vi "Calibration Verifier using Simple State Machine.vi"() -> ()   [LabVIEW 2023]
uses:
  Agilent 3446X Series/Agilent 3446X Series.lvlib
  Keysight E36300 Series/Keysight E36300 Series.lvlib
panel:
  out "error out":errorcluster
  in  "error in":errorcluster
  out "Stabilization":u16(slide) scale=0.0..500.0
  out "Overall Verification":bool
  in  "Test Points & Results":T1(array[cluster])=[{"Volt Set Point (V)"=1.0, "Std Meas (V)"=0.0, "UUT Meas (V)"=0.0, "+/-Delta (V)"=0.1, "Result"=FALSE, "Error (mV)"=0.0}, {"Volt Set Point (V)"=3.3, "Std Meas (V)"=0.0, "UUT Meas (V)"=0.0, "+/-Delta (V)"=0.1, "Result"=FALSE, "Error (mV)"=0.0}, {"Volt Set Point (V)"=5.0, "Std Meas (V)"=0.0, "UUT Meas (V)"=0.0, "+/-Delta (V)"=0.1, "Result"=FALSE, "Error (mV)"=0.0}, {"Volt Set Point (V)"=10.0, "Std Meas (V)"=0.0, "UUT Meas (V)"=0.0, "+/-Delta (V)"=0.1, "Result"=FALSE, "Error (mV)"=0.0}, {"Volt Set Point (V)"=12.0, "Std Meas (V)"=0.0, "UUT Meas (V)"=0.0, "+/-Delta (V)"=0.1, "Result"=FALSE, "Error (mV)"=0.0}]
  # "Multimeter Calibration Verifier"
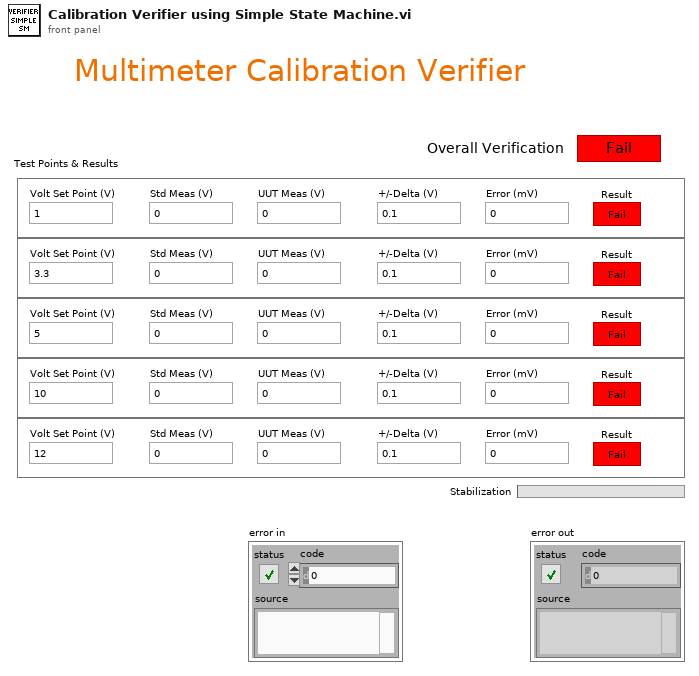
[diagram p1: front panel]
types:
  T1 = cluster{"Volt Set Point (V)":dbl, "Std Meas (V)":dbl, "UUT Meas (V)":dbl, "+/-Delta (V)":dbl, "Result":bool, "Error (mV)":dbl}[]
  T2 = enum16{"Start Calibration", "Set Volt to Power Supply", "Wait for stability", "Dialog Input UUT Meas", "Measure DMM", "Check Limits", "Update Overall Result", "Save Report"}
  T3 = cluster{"Volt Set Point (V)":dbl, "Std Meas (V)":dbl, "UUT Meas (V)":dbl, "+/-Delta (V)":dbl, "Result":bool, "Error (mV)":dbl}
  T4 = typedef "imagedata.ctl" = cluster{"image type":i32, "image depth":i32, "image":u8[], "mask":u8[], "colors":u32[], "Rectangle":cluster{"left":i16, "top":i16, "right":i16, "bottom":i16}}
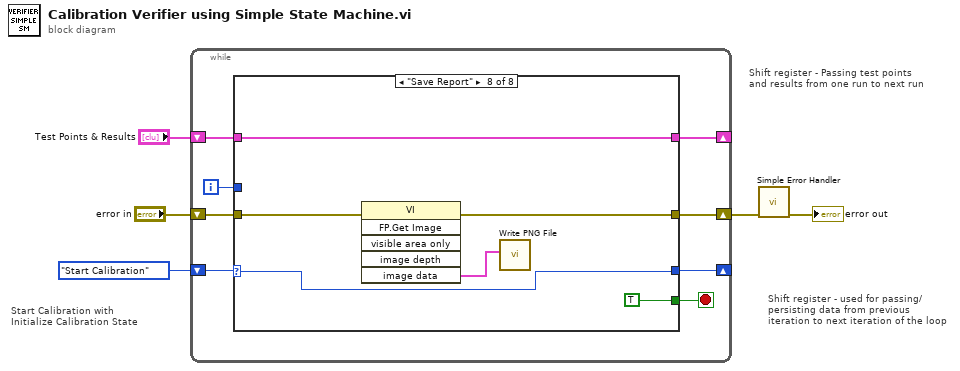
[diagram p0: block diagram]
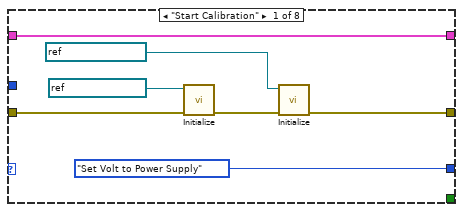
[diagram p2: hidden frame]
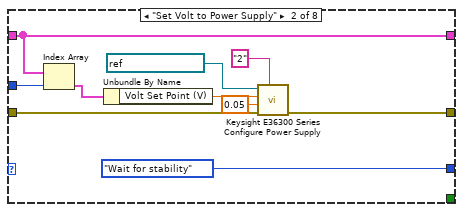
[diagram p3: hidden frame]
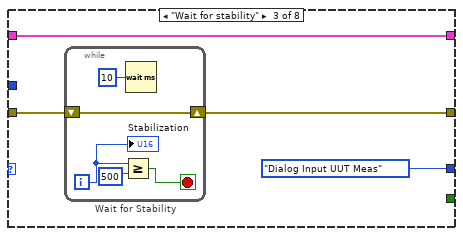
[diagram p4: hidden frame]
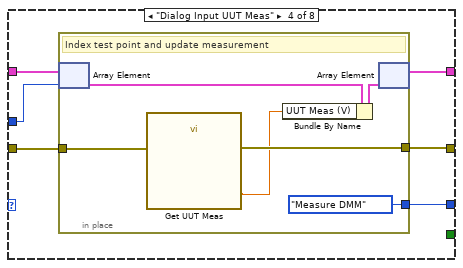
[diagram p5: hidden frame]
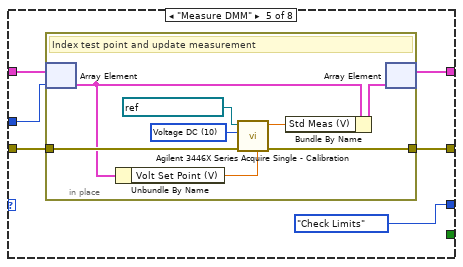
[diagram p6: hidden frame]
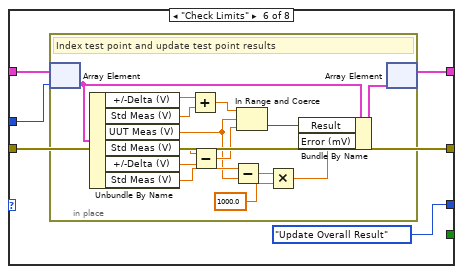
[diagram p7: hidden frame]
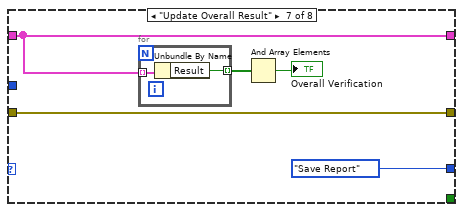
[diagram p8: hidden frame]
diagram:
  # "Shift register - Passing test points and results from one run to next run"
  # "Shift register - used for passing/persisting data from previous iteration to next iteration of the loop"
  # "Start Calibration with  Initialize Calibration State"
  n1 = while {
    shift-right: [w13] -> w4
    shift-left: "error in" -> [w12]
    shift-right: [w8] -> _
    shift-left: "Test Points & Results" -> [w7]
    shift-right: [w10] -> _
    shift-left: T2."Start Calibration" -> [w11]
    i -> [w6]
    stop <- w9 stop-if-true
    n2 = case shown="\"Save Report\"" w11 {
      selector: w11 -> [_ _ _ _ _ _ _ w95]
      tunnel: [w19 w24 w34 w44 w56 w70 w85 w92] -> w13
      tunnel: w12 -> [w18 w30 w31 w45 w57 w70 w85 w93]
      tunnel: [T2."Set Volt to Power Supply" T2."Wait for stability" T2."Dialog Input UUT Meas" w43 T2."Check Limits" T2."Update Overall Result" T2."Save Report" w95] -> w10
      tunnel: [_ _ _ _ _ _ _ TRUE] -> w9
      tunnel: w7 -> [w17 w23 w33 w42 w53 w68 w87 w96]
      tunnel: [w17 w23 w33 w40 w52 w67 w87 w96] -> w8
      tunnel: w6 -> [_ w22 _ w41 w54 w66 _ _]
      frame "Start Calibration" {
        n3 = call "Initialize.vi"("error in (no error)"=w18, "VISA resource name"=refnum<visa-resource-name> "E36312A_PSU") -> ("error out"=w20:errorcluster)  [unwired: 8 in, 1 out]
        n4 = call "Initialize.vi"("error in (no error)"=w20, "VISA resource name"=refnum<visa-resource-name> "34465A_DMM") -> ("error out"=w19:errorcluster)  [unwired: 8 in, 1 out]
      }
      frame "Set Volt to Power Supply" {
        n5 = Index Array(array=w23, index=w22) -> (element=w21:T3)
        n6 = Unbundle By Name(w21) -> ("Volt Set Point (V)"=w27:dbl)
        n7 = call "Keysight E36300 Series Configure Power Supply.vi"("Channel (1)"="2", "error in (no error)"=w30, "Current Level (2 A)"=0.05, "Voltage Level (1 V)"=w27, "VISA resource name"=refnum<visa-resource-name> "E36312A_PSU") -> ("error out"=w24:errorcluster)  [unwired: 6 in]
      }
      frame "Wait for stability" {
        n8 = while "Wait for Stability" {
          shift-right: [w35] -> w34
          shift-left: w31 -> [w35]
          i -> [w38]
          stop <- w36 stop-if-true
          n9 = Greater Or Equal?(x=w38, y=500) -> (x >= y?=w36:bool)
          n10 = Wait (ms)(milliseconds to wait=u32 10) -> ()  [unwired: 1 out]
          "Stabilization" <- w38
        }
      }
      frame "Dialog Input UUT Meas" {
        n11 = in-place {
          in-place-border: w45 -> [w51]
          in-place-border: [w50] -> w44
          in-place-border: [T2."Measure DMM"] -> w43
          # "Index test point and update measurement"
          n12 = in-place-array #1(w42, w41) -> (w46:T3)
          n13 = call "Get UUT Meas"("error in (no error)"=w51) -> ("Voltage (V)"=w49:dbl, "error out"=w50:errorcluster)  [unwired: 16 in, 1 out]
          n14 = Bundle By Name(cluster=w46, "UUT Meas (V)"=w49) -> (w47:T3)
          n15 = in-place-array #1(w47) -> (w40:T1)  [unwired: 1 out]
        }
      }
      frame "Measure DMM" {
        n16 = in-place {
          in-place-border: w57 -> [w65]
          in-place-border: [w64] -> w56
          w63 = 10 items=["Continuity", "Current AC", "Current DC", "Diode", "Frequency", "Resistance 4-wire", "Period", "Resistance 2-wire", "Temperature", "Voltage AC", "Voltage DC", "Voltage DC Ratio", "Capacitance"] ("Measurement Function (10: Voltage DC)")
          # "Index test point and update measurement"
          n17 = in-place-array #2(w53, w54) -> (w59:T3)
          n18 = Unbundle By Name(w59) -> ("Volt Set Point (V)"=w62:dbl)
          n19 = call "Agilent 3446X Series Acquire Single - Calibration.vi"("Sim. Volt Set Point (V)"=w62, "error in (no error)"=w65, "Measurement Function (10: Voltage DC)"=w63, "VISA resource name"=refnum<visa-resource-name> "34465A_DMM") -> ("error out"=w64:errorcluster, "Measurement"=w61:dbl)  [unwired: 6 in]
          n20 = Bundle By Name(cluster=w59, "Std Meas (V)"=w61) -> (w58:T3)
          n21 = in-place-array #2(w58) -> (w52:T1)  [unwired: 1 out]
        }
      }
      frame "Check Limits" {
        n22 = in-place {
          # "Index test point and update test point results"
          n23 = in-place-array #3(w68, w66) -> (w72:T3)
          n24 = Unbundle By Name(w72) -> ("+/-Delta (V)"=w84:dbl, "Std Meas (V)"=w83:dbl, "UUT Meas (V)"=w75:dbl, "Std Meas (V)"=w81:dbl, "+/-Delta (V)"=w82:dbl, "Std Meas (V)"=w76:dbl)
          n25 = Add(x=w84, y=w83) -> (x+y=w80:dbl)
          n26 = Subtract(x=w81, y=w82) -> (x-y=w79:dbl)
          n27 = Subtract(x=w76, y=w75) -> (x-y=w74:dbl)
          n28 = In Range and Coerce(upper limit=w80, x=w75, lower limit=w79) -> (In Range?=w78:bool)  [unwired: 1 out]
          n29 = Multiply(x=w74, y=1000.0) -> (x*y=w73:dbl)
          n30 = Bundle By Name(cluster=w72, "Result"=w78, "Error (mV)"=w73) -> (w71:T3)
          n31 = in-place-array #3(w71) -> (w67:T1)  [unwired: 1 out]
        }
      }
      frame "Update Overall Result" {
        n32 = for {
          tunnel: w87 -> [w91] mode=indexing
          tunnel: [w90] -> w88 mode=indexing
          n33 = Unbundle By Name(w91) -> ("Result"=w90:bool)
        }
        n34 = And Array Elements(Boolean array=w88) -> (logical AND=→"Overall Verification":bool)
      }
      frame "Save Report" {
        n35 = invoke class="VI" method="FP.Get Image"(error in=w93) -> (error out=w92:errorcluster, "image data"=w94:T4)  [unwired: 5 in, 4 out]
        n36 = call <vilib>:"Write PNG File.vi"("image data"=w94) -> ()  [unwired: 9 in, 2 out]
      }
    }
  }
  n37 = call <vilib>:"Simple Error Handler.vi"("error in (no error)"=w4) -> ("error out"=→"error out":errorcluster)  [unwired: 4 in, 4 out]
